vi "_PC_Pub_FM stateMachine.vi"(7 "Func":T1, 8 "error in (no error)":errorcluster, 9 "elementData":waveform(sgl), 10 "timeStamp":string, 11 "tdmsFilePath in":path) -> (0 "error out":errorcluster, 2 "outputDataArray":string[][](array[string]), 3 "tdmsFilePath out":path)   [LabVIEW 2018, in "FM.lvclass"]
uses:
  FM.lvclass
  ctl/_PC_Pub_FM stateMachineEnum.ctl
  ctl/_PC_Pub_FM fileReadFuncEnum.ctl
  <vilib>/Utility/error.llb/Error Cluster From Error Code.vi
  <vilib>/ErrorRing/Error Ring.xnode
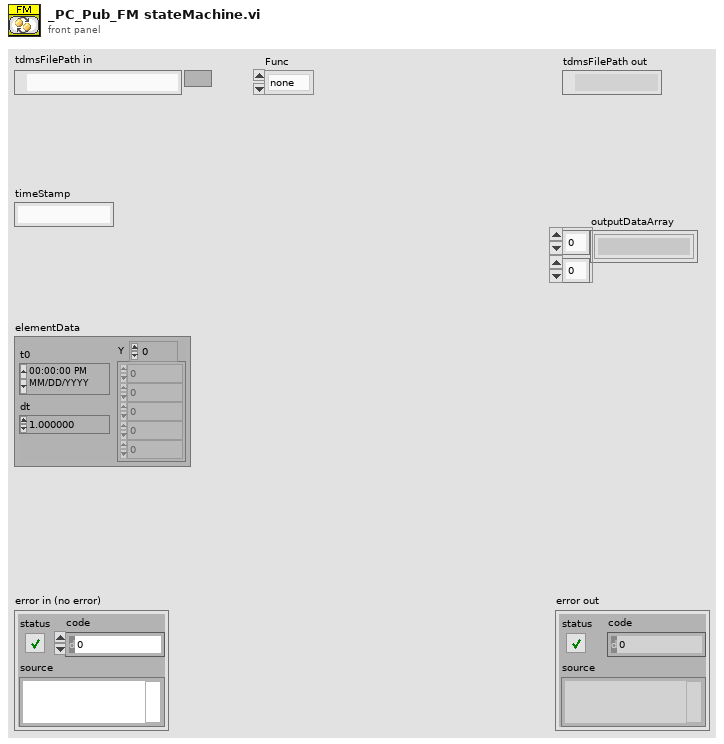
[diagram p1: front panel]
types:
  T1 = typedef "_PC_Pub_FM stateMachineEnum.ctl" = enum16{"none", "init", "reset_t0", "openTDMS", "writeTDMS", "closeTDMS", "readTDMS", "getDataItems"}
  T2 = enum16{"open", "open or create", "create or replace", "create", "open (read-only)"}
  T3 = typedef "_PC_Pub_FM fileReadFuncEnum.ctl" = enum16{"getAllInfo", "getChromatogram", "getDataItems", "getTimeStamp", "getIdxData", "getIonization", "getRemark", "getAttrFormat"}
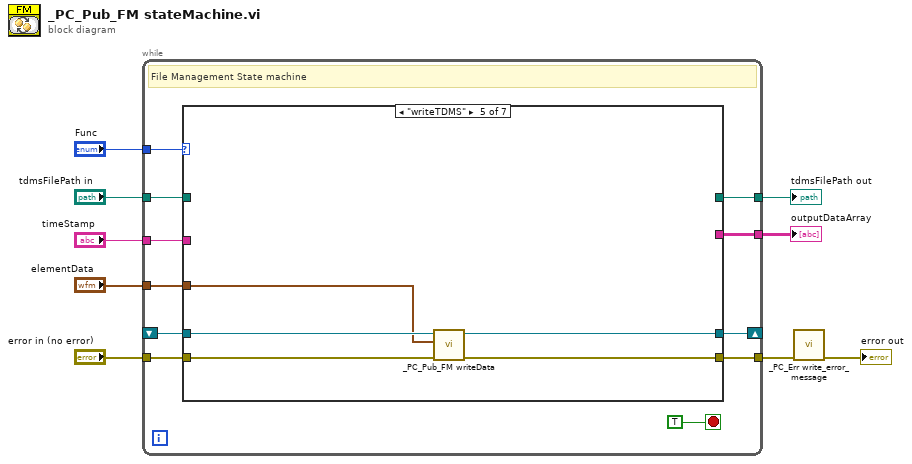
[diagram p0: block diagram]
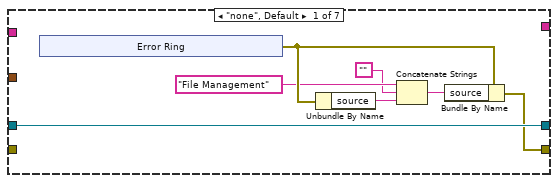
[diagram p2: hidden frame]
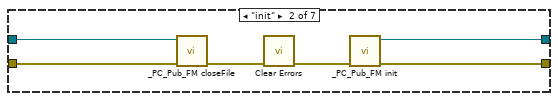
[diagram p3: hidden frame]
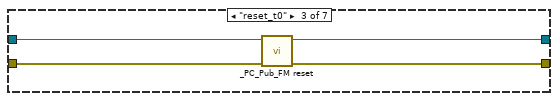
[diagram p4: hidden frame]
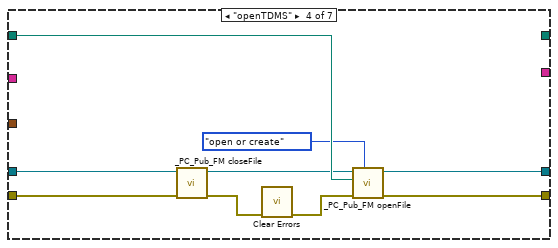
[diagram p5: hidden frame]
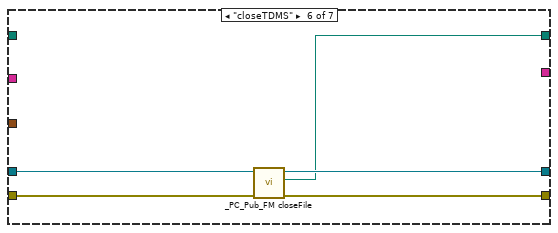
[diagram p6: hidden frame]
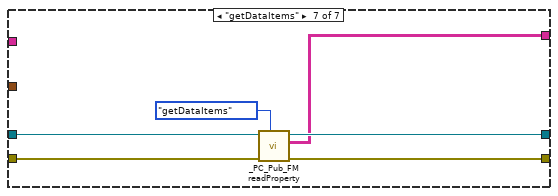
[diagram p7: hidden frame]
diagram:
  n1 = while {
    tunnel: "Func" -> [w19]
    shift-right: [w18] -> _
    shift-left: _ -> [w17]
    tunnel: [w16] -> w9
    tunnel: "error in (no error)" -> [w15]
    tunnel: "tdmsFilePath in" -> [w14]
    tunnel: [w13] -> w4
    tunnel: "timeStamp" -> [w12]
    tunnel: [w11] -> w2
    tunnel: "elementData" -> [w10]
    stop <- TRUE stop-if-true
    # "File Management State machine"
    n2 = case shown="\"writeTDMS\"" w19 {
      tunnel: [w27 w37 w40 w50 w52 w57 w63] -> w18
      tunnel: w17 -> [w27 w36 w41 w47 w55 w60 w66]
      tunnel: [w21 w33 w39 w49 w53 w58 w64] -> w16
      tunnel: w15 -> [_ w32 w38 w46 w54 w59 w65]
      tunnel: w14 -> [_ _ _ w48 _ _ _]
      tunnel: [_ _ _ _ _ w56 _] -> w13
      tunnel: w12 -> [_ _ _ _ _ _ _]
      tunnel: [_ _ _ _ _ _ w62] -> w11
      tunnel: w10 -> [_ _ _ _ w51 _ _]
      frame "none", Default {
        n3 = xnode "Error Ring"() -> ("error out"=w24:errorcluster)
        n4 = Unbundle By Name(w24) -> ("source"=w25:string)
        n5 = Concatenate Strings("File Management" ("string"), "", w25) -> (w26:string)
        n6 = Bundle By Name(cluster=w24, "source"=w26) -> (w21:errorcluster)
      }
      frame "init" {
        n7 = call "_PC_Pub_FM closeFile.vi"("error in (no error)"=w32, "FM in"=w36) -> ("error out"=w35:errorcluster)  [unwired: 7 in, 2 out]
        n8 = call <vilib>:"Clear Errors.vi"("error in (no error)"=w35) -> ("error out"=w34:errorcluster)  [unwired: 5 in, 1 out]
        n9 = call "_PC_Pub_FM init.vi"("error in (no error)"=w34) -> ("error out"=w33:errorcluster, "FM out"=w37:refnum<class "FM.lvclass">)  [unwired: 9 in]
      }
      frame "reset_t0" {
        n10 = call "_PC_Pub_FM reset.vi"("error in (no error)"=w38, "FM in"=w41) -> ("error out"=w39:errorcluster, "FM out"=w40:refnum<class "FM.lvclass">)  [unwired: 8 in]
      }
      frame "openTDMS" {
        n11 = call "_PC_Pub_FM closeFile.vi"("error in (no error)"=w46, "FM in"=w47) -> ("error out"=w45:errorcluster, "FM out"=w43:refnum<class "FM.lvclass">)  [unwired: 7 in, 1 out]
        n12 = call <vilib>:"Clear Errors.vi"("error in (no error)"=w45) -> ("error out"=w44:errorcluster)  [unwired: 5 in, 1 out]
        n13 = call "_PC_Pub_FM openFile.vi"("operation (0:open)"=T2."open or create", "error in (no error)"=w44, "openPath"=w48, "FM in"=w43) -> ("error out"=w49:errorcluster, "FM out"=w50:refnum<class "FM.lvclass">)  [unwired: 6 in]
      }
      frame "writeTDMS" {
        n14 = call "_PC_Pub_FM writeData.vi"("error in (no error)"=w54, "element"=w51, "FM in"=w55) -> ("error out"=w53:errorcluster, "FM out"=w52:refnum<class "FM.lvclass">)  [unwired: 7 in]
      }
      frame "closeTDMS" {
        n15 = call "_PC_Pub_FM closeFile.vi"("error in (no error)"=w59, "FM in"=w60) -> ("error out"=w58:errorcluster, "filePath"=w56:path, "FM out"=w57:refnum<class "FM.lvclass">)  [unwired: 7 in]
      }
      frame "getDataItems" {
        n16 = call "_PC_Pub_FM readProperty.vi"("readEvent"=_PC_Pub_FM_fileReadFuncEnum."getDataItems", "error in (no error)"=w65, "FM in"=w66) -> ("error out"=w64:errorcluster, "outputArr"=w62:string[][], "FM out"=w63:refnum<class "FM.lvclass">)  [unwired: 6 in]
      }
    }
  }
  "tdmsFilePath out" <- w4
  "outputDataArray" <- w2
  n17 = call "_PC_Err write_error_message.vi"("error in"=w9) -> ("error out"=→"error out":errorcluster)  [unwired: 10 in]
